vi "Convert_Graph_v00.vi"(8 "Extras PII":T1, 11 "PII Control":T2={"Offset Error"=-0.08983050847457627, "Gain Error"=1, "P Gain"=0, "P Bit Shift"=1, "I Bit Shift"=20, "I2 Bit Shift"=-12, "I Gain"=-12, "I2 Gain"=-27, "Lock Threshold"=20, "Lock"=FALSE, "Hold"=FALSE, "Scan Frequency"=8, "Scan Bit Shift"=-5, "Gains -ve "=TRUE, "Pre- Offset Error"=-4.0} {"Pre- Offset Error" scale=-0.01..0.01 scale format="%#_5f"; "Scan Frequency" scale=1.0..30.0; "I2 Gain" scale=0.0..10.0; "I Gain" scale=0.0..50.0; "P Gain" scale=0.0..50.0; "Offset Error" scale=-0.01..0.01 scale format="%#_5f"}) -> (3 "PII+Error":T11)   [LabVIEW 2010]
uses:
  Strict Type Defs/PII individual.ctl
  Strict Type Defs/Errors Converted Graph.ctl
  Strict Type Defs/PII and Error Graph.ctl
  Strict Type Defs/Control GUI Graph v00.ctl
  Strict Type Defs/Slider and display.ctl
  Strict Type Defs/I16 white control.ctl
  Strict Type Defs/PII Gains.ctl
  Strict Type Defs/I2 gain slider.ctl
  Strict Type Defs/Thresh slider.ctl
  Strict Type Defs/Lock or Hold.ctl
  Strict Type Defs/Scan Freq Slider.ctl
  Strict Type Defs/Gains negative vertical.ctl
  Strict Type Defs/Extras PII Graph.ctl
panel:
  in  "PII+Error":T11
  in  "Error individual":T12
  in  "PII In typdef":T13
  # "PII Gains"
  # "Lock"
  # "Error Signal"
  # "Scan"
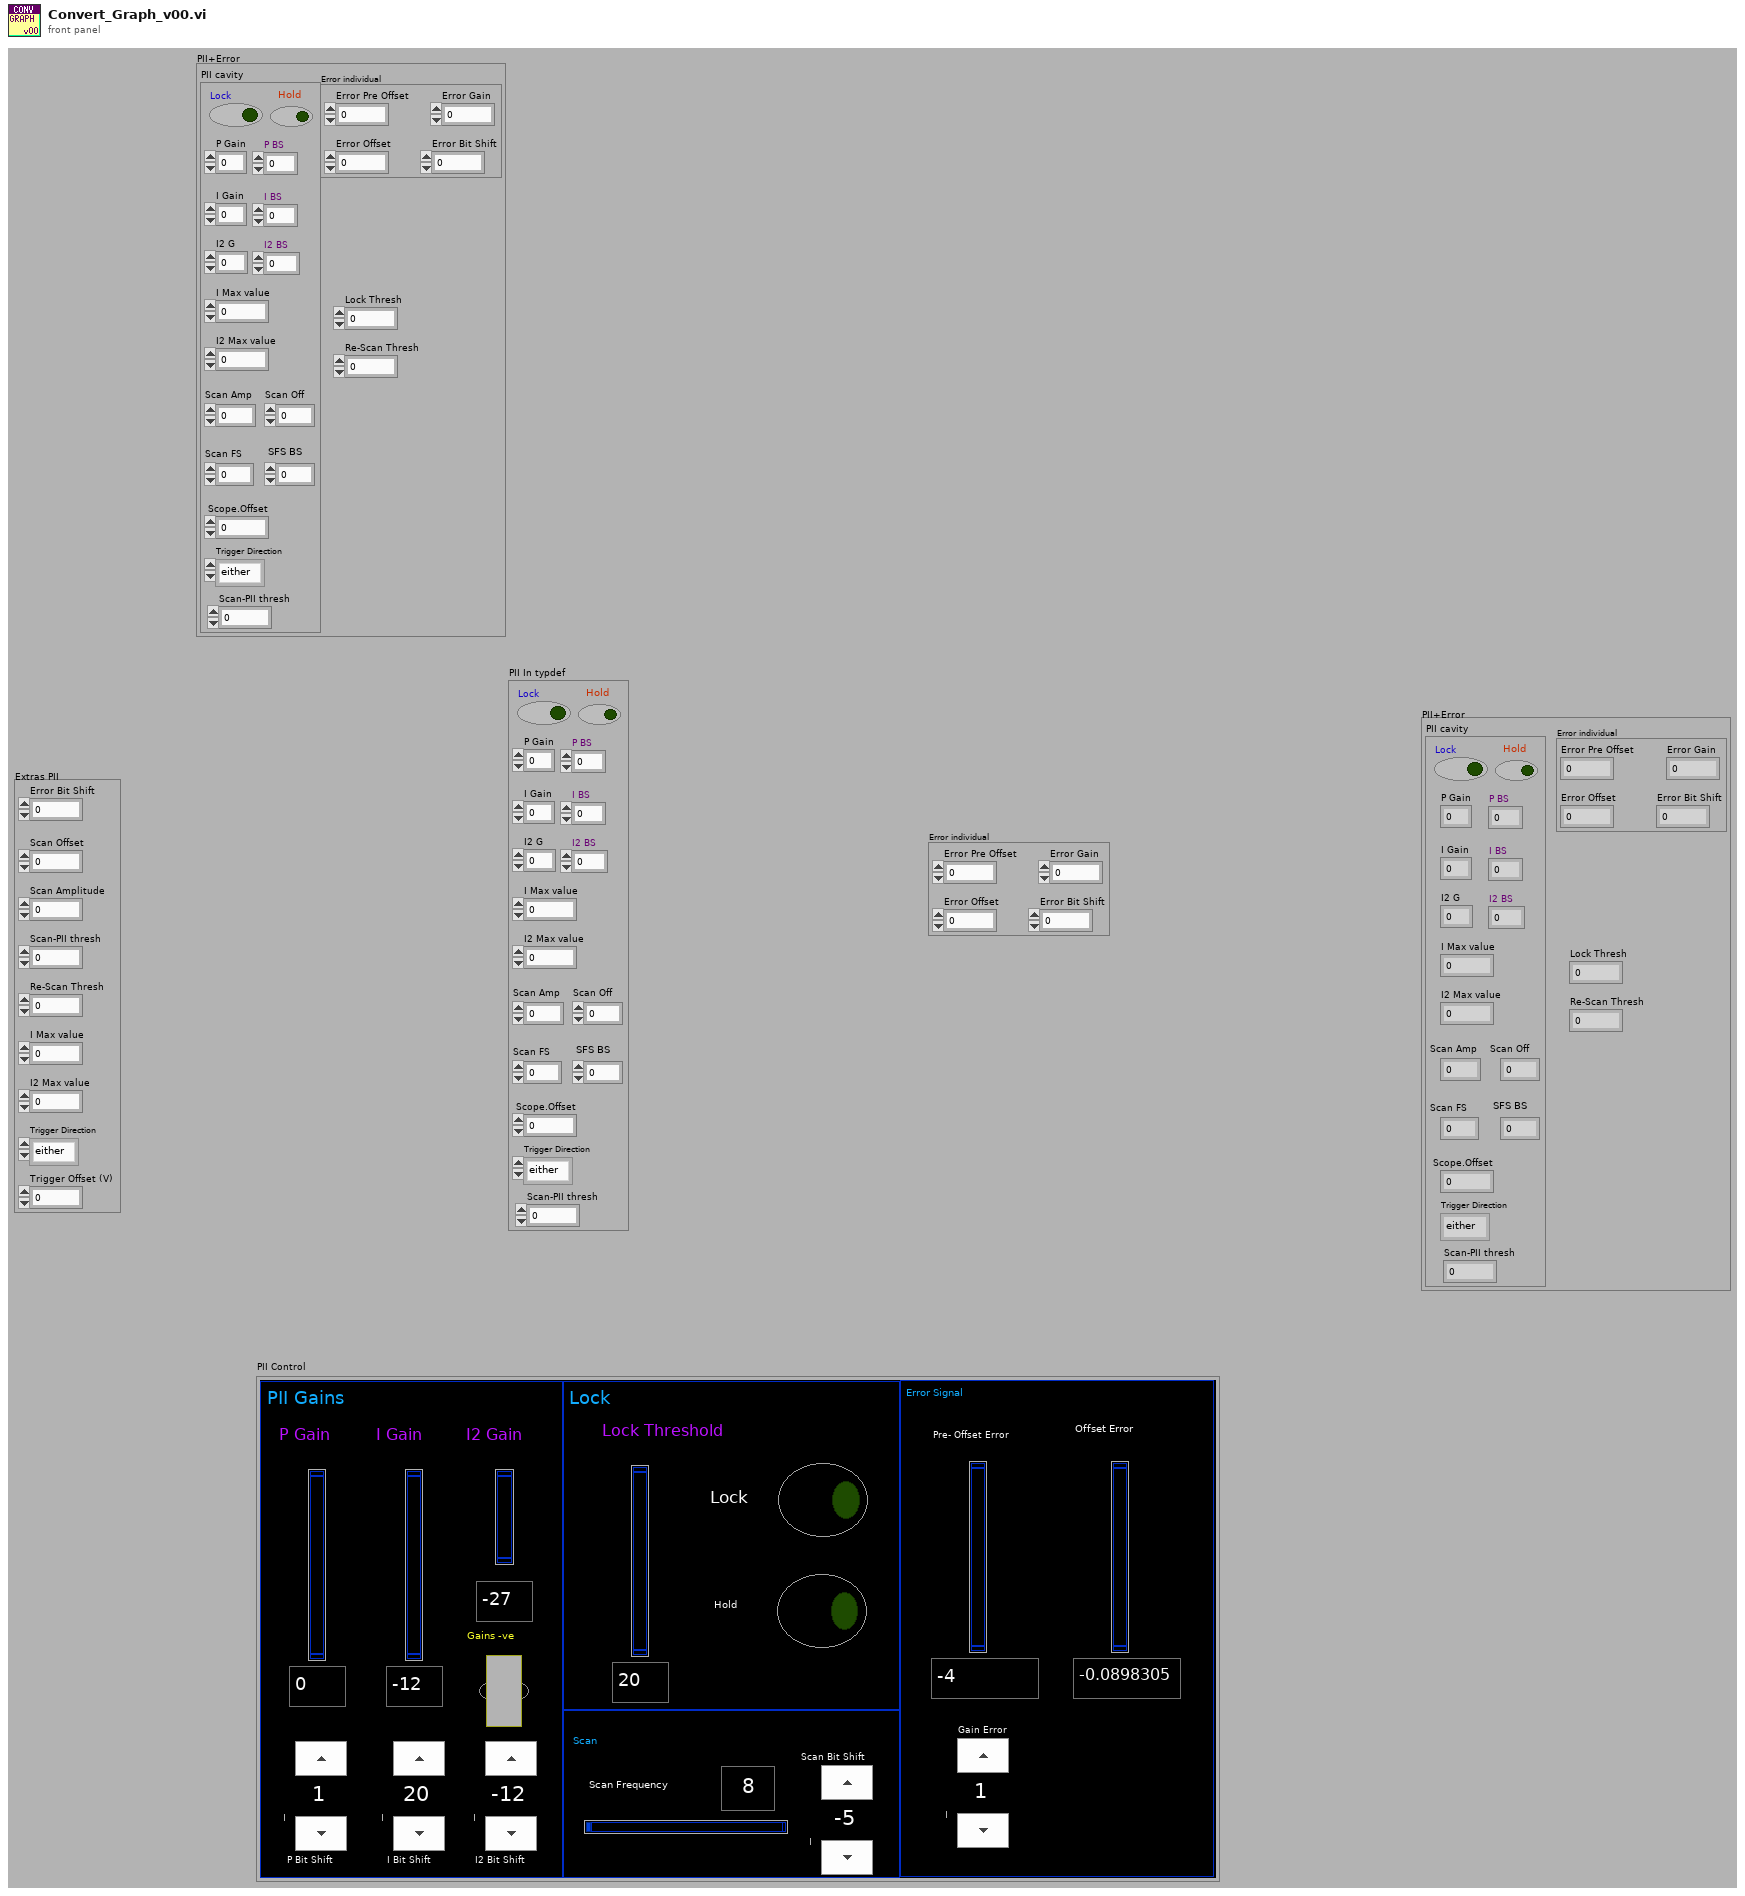
[diagram p1: front panel]
types:
  T1 = typedef "Extras PII Graph.ctl" = cluster{"Error Bit Shift":i16, "Scan Offset":dbl, "Scan Amplitude":dbl, "Scan-PII thresh":i16, "Re-Scan Thresh":i16, "I Max value":i32, "I2 Max value":i32, "Trigger Direction":enum8{"either", "minus-plus", "plus-minus"}, "Trigger Offset (V)":dbl}
  T2 = typedef "Control GUI Graph v00.ctl" = cluster{"Offset Error":T3, "Gain Error":T4, "P Gain":T5, "P Bit Shift":T4, "I Bit Shift":T4, "I2 Bit Shift":T4, "I Gain":T5, "I2 Gain":T6, "Lock Threshold":T7, "Lock":T8, "Hold":T8, "Scan Frequency":T9, "Scan Bit Shift":T4, "Gains -ve ":T10, "Pre- Offset Error":T3}
  T3 = typedef "Slider and display.ctl" = dbl
  T4 = typedef "I16 white control.ctl" = i16
  T5 = typedef "PII Gains.ctl" = i32
  T6 = typedef "I2 gain slider.ctl" = i32
  T7 = typedef "Thresh slider.ctl" = i16
  T8 = typedef "Lock or Hold.ctl" = bool
  T9 = typedef "Scan Freq Slider.ctl" = u16
  T10 = typedef "Gains negative vertical.ctl" = bool
  T11 = typedef "PII and Error Graph.ctl" = cluster{"Error individual":T12, "PII cavity":T13, "Lock Thresh":i16, "Re-Scan Thresh":i16}
  T12 = typedef "Errors Converted Graph.ctl" = cluster{"Error Pre Offset":i16, "Error Offset":i16, "Error Gain":i16, "Error Bit Shift":i16}
  T13 = typedef "PII individual.ctl" = cluster{"Lock":bool, "Hold":bool, "P Gain":i32, "P BS":i16, "I Gain":i32, "I BS":i16, "I2 G":i32, "I2 BS":i16, "Scan Amp":i16, "Scan Off":i16, "Scan FS":u16, "SFS BS":i16, "I Max value":i32, "I2 Max value":i32, "Scope.Offset":i16, "Trigger Direction":enum8{"either", "minus-plus", "plus-minus"}, "Scan-PII thresh":i16}
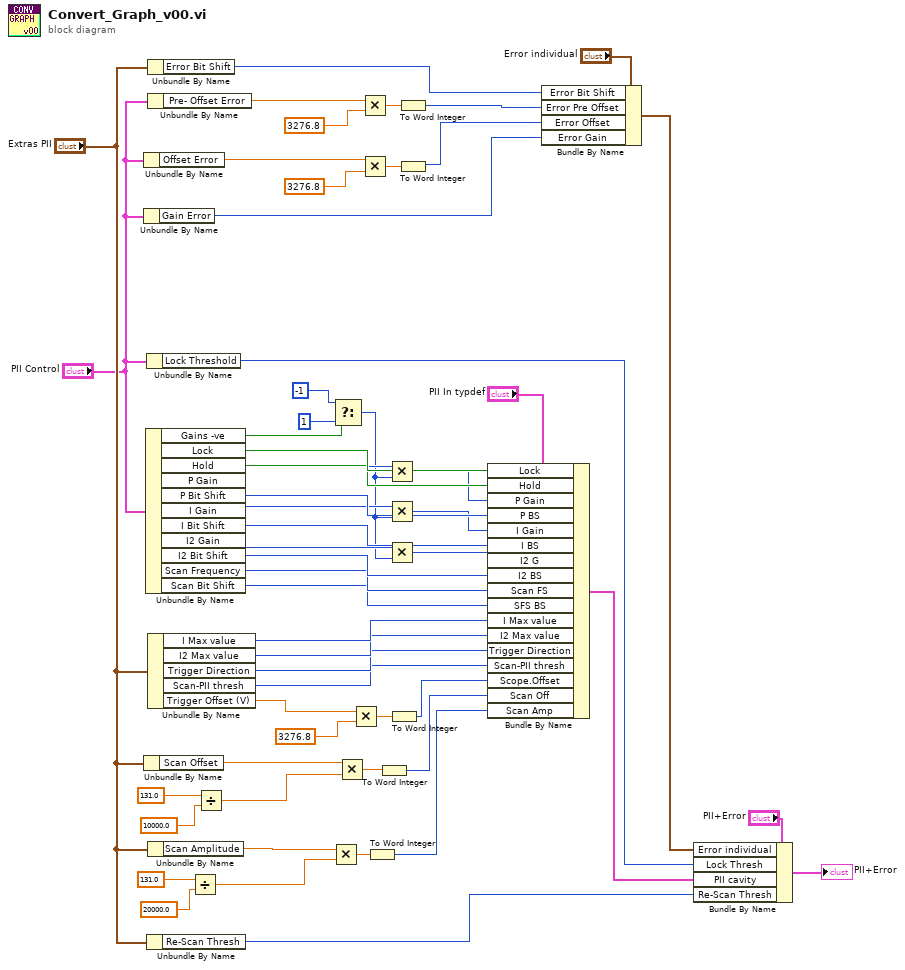
[diagram p0: block diagram]
diagram:
  n1 = Unbundle By Name("PII Control") -> ("Offset Error"=w53:T3)
  n2 = Unbundle By Name("PII Control") -> ("Gain Error"=w20:T4)
  n3 = Unbundle By Name("Extras PII") -> ("Scan Offset"=w18:dbl)
  n4 = Unbundle By Name("PII Control") -> ("Gains -ve"=w37:T10, "Lock"=w42:T8, "Hold"=w41:T8, "P Gain"=w36:T5, "P Bit Shift"=w40:T4, "I Gain"=w32:T5, "I Bit Shift"=w39:T4, "I2 Gain"=w30:T6, "I2 Bit Shift"=w38:T4, "Scan Frequency"=w27:T9, "Scan Bit Shift"=w26:T4)
  n5 = Unbundle By Name("PII Control") -> ("Lock Threshold"=w17:T7)
  n6 = Unbundle By Name("Extras PII") -> ("Re-Scan Thresh"=w5:i16)
  n7 = Unbundle By Name("Extras PII") -> ("Error Bit Shift"=w1:i16)
  n8 = Unbundle By Name("PII Control") -> ("Pre- Offset Error"=w2:T3)
  n9 = Unbundle By Name("Extras PII") -> ("I Max value"=w14:i32, "I2 Max value"=w13:i32, "Trigger Direction"=w12:enum8{"either", "minus-plus", "plus-minus"}, "Scan-PII thresh"=w11:i16, "Trigger Offset (V)"=w7:dbl)
  n10 = Unbundle By Name("Extras PII") -> ("Scan Amplitude"=w52:dbl)
  n11 = Divide(x=131.0, y=20000.0) -> (x/y=w47:dbl)
  n12 = Divide(x=131.0, y=10000.0) -> (x/y=w44:dbl)
  n13 = Multiply(x=w52, y=w47) -> (x*y=w50:dbl)
  n14 = Select(t=T5 -1 ("y"), s=w37, f=T5 1) -> (s? t:f=w28:T5)
  n15 = Multiply(x=w18, y=w44) -> (x*y=w51:dbl)
  n16 = Multiply(x=w7, y=3276.8) -> (x*y=w9:dbl)
  n17 = Multiply(x=w2, y=3276.8) -> (x*y=w56:T3)
  n18 = Multiply(x=w53, y=3276.8) -> (x*y=w55:T3)
  n19 = To Word Integer(number=w50) -> (16bit integer=w16:i16)
  n20 = To Word Integer(number=w51) -> (16bit integer=w10:i16)
  n21 = Multiply(x=w36, y=w28) -> (x*y=w33:T5)
  n22 = Multiply(x=w32, y=w28) -> (x*y=w31:T5)
  n23 = Multiply(x=w30, y=w28) -> (x*y=w29:T6)
  n24 = To Word Integer(number=w9) -> (16bit integer=w6:i16)
  n25 = To Word Integer(number=w56) -> (16bit integer=w24:i16)
  n26 = To Word Integer(number=w55) -> (16bit integer=w23:i16)
  n27 = Bundle By Name(cluster="PII In typdef", "Lock"=w42, "Hold"=w41, "P Gain"=w33, "P BS"=w40, "I Gain"=w31, "I BS"=w39, "I2 G"=w29, "I2 BS"=w38, "Scan FS"=w27, "SFS BS"=w26, "I Max value"=w14, "I2 Max value"=w13, "Trigger Direction"=w12, "Scan-PII thresh"=w11, "Scope.Offset"=w6, "Scan Off"=w10, "Scan Amp"=w16) -> (w21:T13)
  n28 = Bundle By Name(cluster="Error individual", "Error Bit Shift"=w1, "Error Pre Offset"=w24, "Error Offset"=w23, "Error Gain"=w20) -> (w4:T12)
  n29 = Bundle By Name(cluster="PII+Error", "Error individual"=w4, "Lock Thresh"=w17, "PII cavity"=w21, "Re-Scan Thresh"=w5) -> (→"PII+Error":T11)
